vi "Load Packed Library.vi"(8 "error in (no error)":errorcluster, 10 "packed library name":string, 11 "Component Loader in":refnum<class "Component Loader.lvclass">) -> (0 "error out":errorcluster, 2 "objects":refnum<class>[](array[class]), 3 "Component Loader out":refnum<class "Component Loader.lvclass">)   [LabVIEW 2019, in "DSF Core.lvlib" / "Component Loader.lvclass"]
uses:
  Component Loader.lvclass
  Component Loader.lvclass/Component Loader.ctl
  Find Packed Libraries.vi
  Errors.vi
  Component Not Found.vi
  Load Class.vi
  New Component Loader Error.vi
  <vilib>/NI/Memory Manager/VIs/Write String to Source.vi
  Class Not Found.vi
  <vilib>/NI/Memory Manager/VIs/New Error Cluster.vi
  <vilib>/NI/Memory Manager/VIs/New Error Cluster (512B).vi
  Component Loader Error Info.vi
  <vilib>/NI/Memory Manager/VIs/Set Error Code.vi
  <vilib>/NI/Memory Manager/VIs/Set Error Status.vi
  <vilib>/NI/Memory Manager/VIs/Set Error Source.vi
  VIs/Constants/Constants.vi
  VIs/Constants/Engine Library Name.vi
  Base Error Offset.vi
  VIs/Constants/Base Error Code.vi
  <vilib>/Utility/libraryn.llb/Recursive File List.vi
  <vilib>/Utility/LVLibp/Get Exported File List.vi
  <vilib>/Utility/libraryn.llb/Check if File or Folder Exists.vi
  <vilib>/Utility/LVClass/Get LV Class Default Value.vi
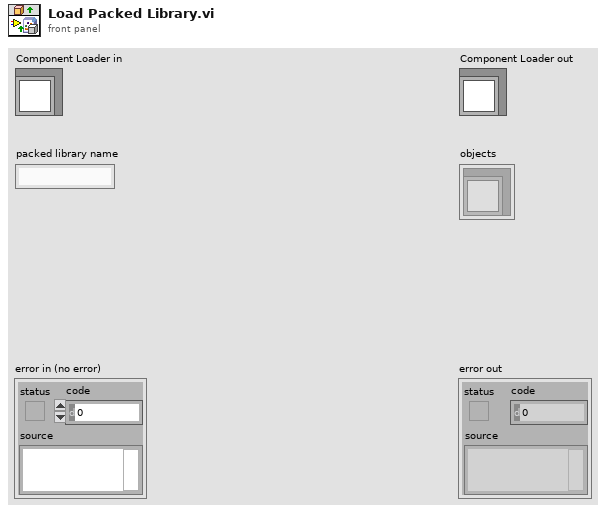
[diagram p1: front panel]
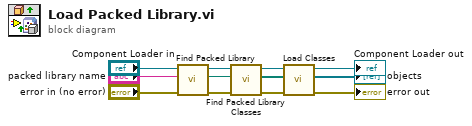
[diagram p0: block diagram]
diagram:
  n1 = call "Find Packed Library.vi"("error in (no error)"="error in (no error)", "packed library name"="packed library name", "Component Loader in"="Component Loader in") -> ("error out"=w8:errorcluster, "packed library path"=w1:path, "Component Loader out"=w9:refnum<class "Component Loader.lvclass">)  [unwired: 6 in]
  n2 = call "Find Packed Library Classes.vi"("error in (no error)"=w8, "packed library path"=w1, "Component Loader in"=w9) -> ("error out"=w6:errorcluster, "class paths"=w5:path[], "Component Loader out"=w7:refnum<class "Component Loader.lvclass">)  [unwired: 6 in]
  n3 = call "Load Classes.vi"("error in (no error)"=w6, "class paths"=w5, "Component Loader in"=w7) -> ("error out"=→"error out":errorcluster, "objects"=→"objects":refnum<class>[], "Component Loader out"=→"Component Loader out":refnum<class "Component Loader.lvclass">)  [unwired: 6 in]
